vi "Init2.vi"(10 "All_info":string[][](array[string])=[["COM", "COM10", "", ""], ["Save Data", "C:\\AC-BarCode\\Save Data\\", "", ""], ["Model", "C:\\AC-BarCode\\Setting Data\\Model.csv", "", ""], ["CheckPars", "3", "4", "5"], ["LINE", "LINE7", "", ""], ["Title", "三部品照合", "", ""], ["sound", "C:\\AC-BarCode\\sound", "", ""], ["ClearTime", "5", "", ""], ["CheckNum", "3", "", ""], ["LotNo", "11:5", "0:8", "11:8"], ["STANO", "1", "1", "1"], ["WORKNO", "壓縮機", "馬達", "電源板"], ["USEQTY", "1", "1", "1"], ["OPUSER", "SYSTEM", "SYSTEM", "SYSTEM"], ["MMODU", "641", "641", "641"]], 11 "DataIn":T2) -> (3 "DataOut":T2)   [LabVIEW 2014]
uses:
  controls/Data1.ctl
  controls/Payjson.ctl
  controls/Pajson.ctl
panel:
  in  "json 2":T1
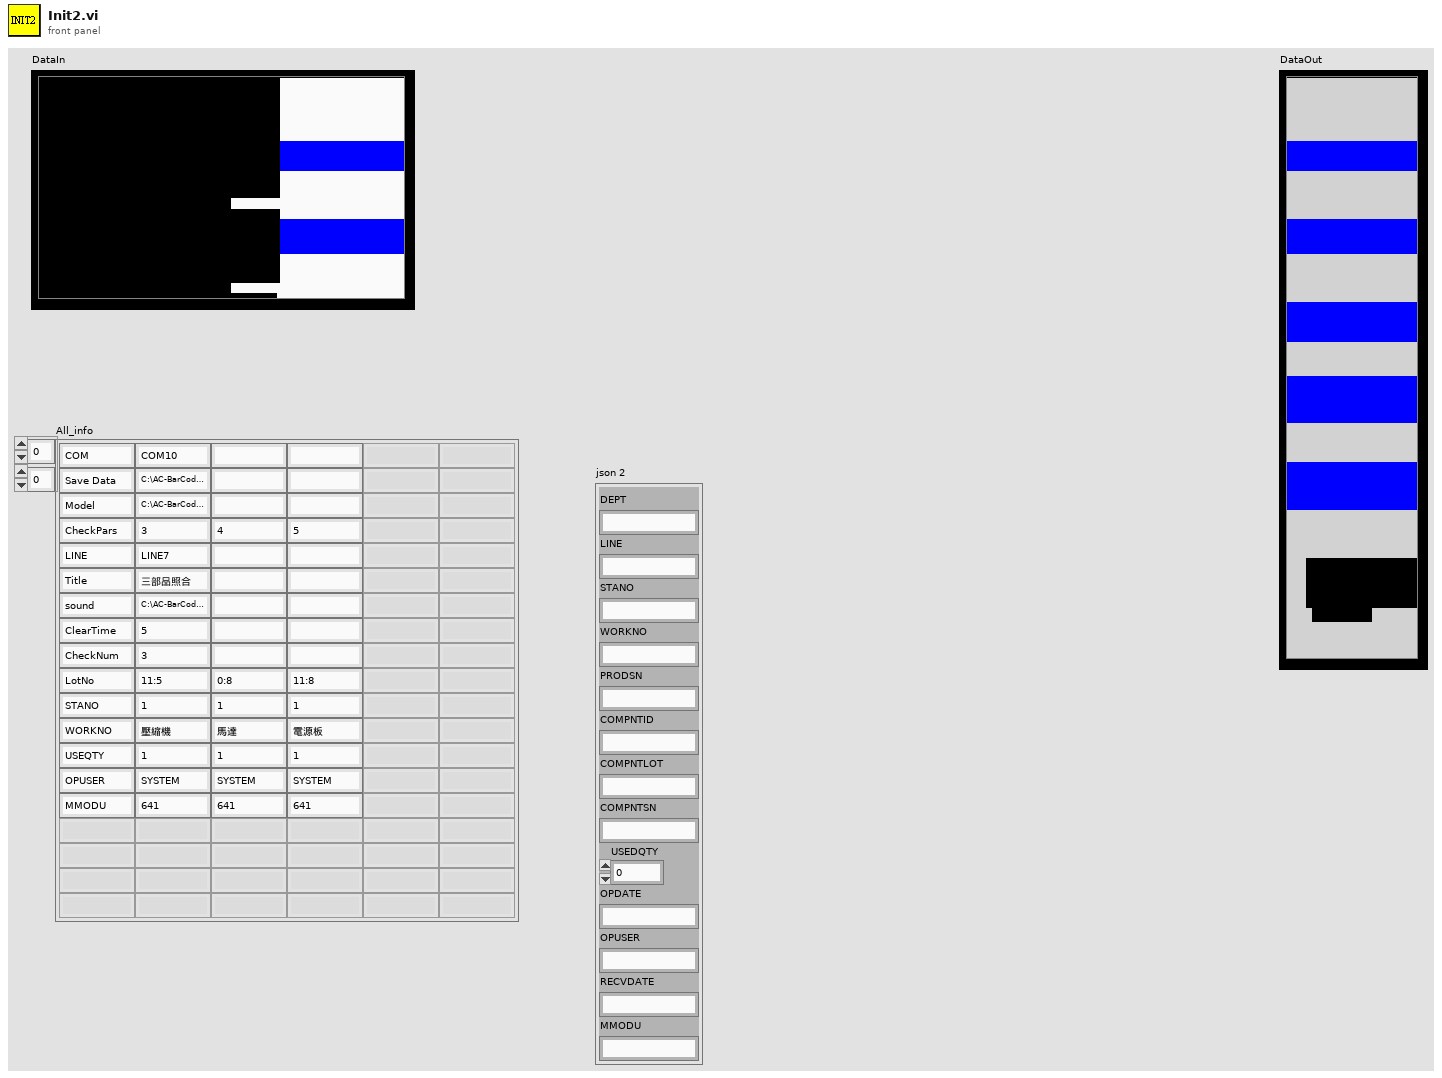
[diagram p1: front panel]
types:
  T1 = typedef "Pajson.ctl" = cluster{"DEPT":string, "LINE":string, "STANO":string, "WORKNO":string, "PRODSN":string, "COMPNTID":string, "COMPNTLOT":string, "COMPNTSN":string, "USEDQTY":i16, "OPDATE":string, "OPUSER":string, "RECVDATE":string, "MMODU":string}
  T2 = typedef "Data1.ctl" = cluster{"Date":string, "BarCode1":string, "BarCode2":string, "BarCode3":string, "Message":string, "OK Count":u16, "NG Count":u16, "Total Count":u16, "ModelData":string[][], "OK&NG":bool, "COM1":refnum<visa-resource-name>, "COM2":refnum<visa-resource-name>, "IO":i32, "Time":u32, "TCP":refnum<k5>, "TCP 2":refnum<k5>, "COM1 2":refnum<visa-resource-name>, "CheckNum":string, "BarCode1_1":string, "BarCode2_1":string, "BarCode3_1":string, "日期":string, "機種":string, "機號":string, "商品條碼1":string, "OK_1":string, "OK":string, "NG":string, "NG_1":string, "Total":string, "Total_1":string, "ClaerTime":u32, "Pjson":T3, "LotNo":string[], "CheckParsArray":string[], "BarCode4":string, "BarCode4_1":string, "商品條碼2":string, "BarCode5":string, "BarCode5_1":string, "商品條碼3":string, "ReScanNG":i32, "NGTimeCT":u32}
  T3 = typedef "Payjson.ctl" = cluster{"DEPT":string, "LINE":string, "STANO":string, "WORKNO":string, "PRODSN":string, "COMPNTID":string, "COMPNTLOT":string, "COMPNTSN":string, "USEDQTY":i16, "OPDATE":string, "OPUSER":string, "RECVDATE":string, "MMODU":string}[]
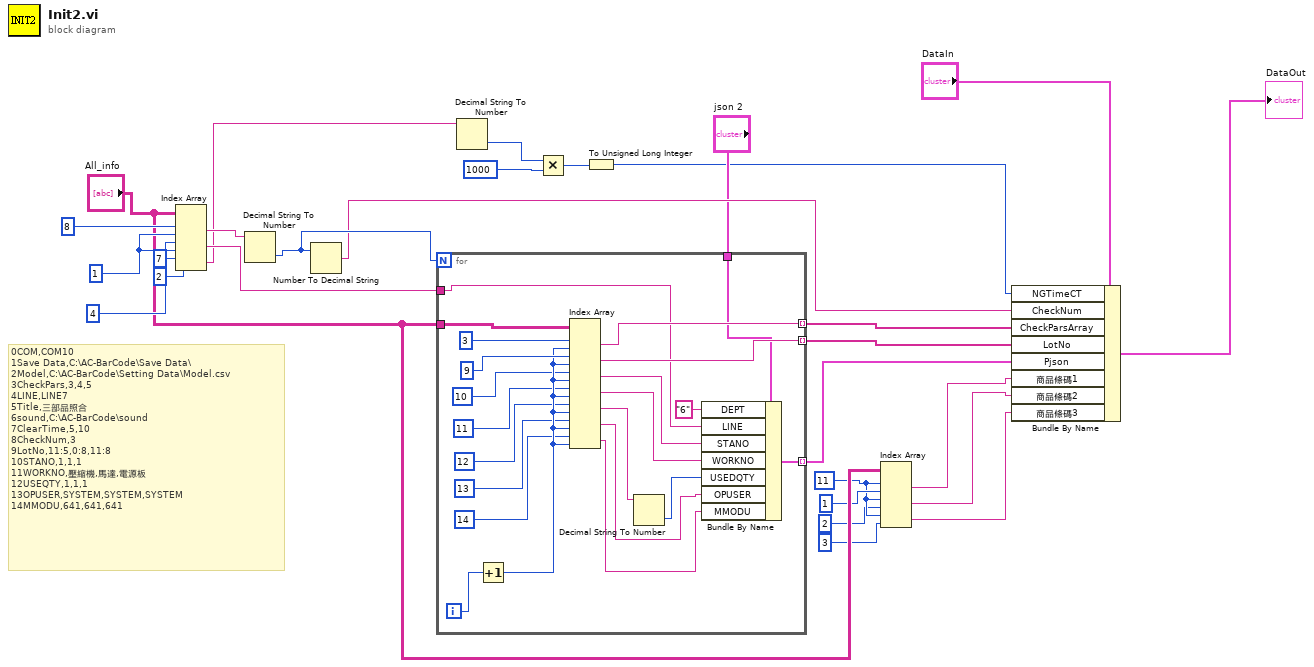
[diagram p0: block diagram]
diagram:
  w13 = 11 ("index (row)")
  w22 = 1 ("disabled index (col)")
  # "0COM,COM10\n1Save Data,C:\\AC-BarCode\\Save Data\\\n2Model,C:\\AC-BarCode\\Setting Data\\Model.csv\n3CheckPars,3,4,5\n4LINE,LINE7\n5Title,三部品照合\n6sound,C:\\AC-BarCode\\sound\n7ClearTime,5,10\n8CheckNum,3\n9LotNo,11:5,0:8,11:8\n10STANO,1,1,1\n11WORKNO,壓縮機,馬達,電源板\n12USEQTY,1,1,1\n13OPUSER,SYSTEM,SYSTEM,SYSTEM\n14MMODU,641,641,641"
  n1 = Index Array(array="All_info", index (row) #1=8 ("disabled index (row)"), index (col) #1=w22, index (row) #2=4 ("disabled index (row)"), index (col) #2=w22, index (row) #3=7 ("index (row)"), index (col) #3=2 ("disabled index (col)")) -> (element #1=w27:string, element #2=w20:string, element #3=w3:string)
  n2 = Decimal String To Number(string=w27) -> (number=w26:i32)  [unwired: 2 in, 1 out]
  n3 = Number To Decimal String(number=w26) -> (decimal integer string=w25:string)  [unwired: 1 in]
  n4 = for {
    N: w26 -> [_]
    tunnel: "All_info" -> [w50]
    tunnel: [w40] -> w24 mode=indexing
    tunnel: [w39] -> w23 mode=indexing
    tunnel: w20 -> [w36]
    tunnel: "json 2" -> [w38]
    tunnel: [w29] -> w18 mode=indexing
    i -> [w49]
    n5 = Increment(x=w49) -> (x+1=w46:i32)
    n6 = Index Array(array=w50, index (row) #1=3 ("disabled index (row)"), index (col) #1=w46, index (row) #2=9 ("disabled index (row)"), index (col) #2=w46, index (row) #3=10 ("disabled index (row)"), index (col) #3=w46, index (row) #4=11 ("disabled index (row)"), index (col) #4=w46, index (row) #5=12 ("disabled index (row)"), index (col) #5=w46, index (row) #6=13 ("disabled index (row)"), index (col) #6=w46, index (row) #7=14 ("disabled index (row)"), index (col) #7=w46) -> (element #1=w40:string, element #2=w39:string, element #3=w35:string, element #4=w34:string, element #5=w33:string, element #6=w31:string, element #7=w30:string)
    n7 = Decimal String To Number(string=w33) -> (number=w32:i32)  [unwired: 2 in, 1 out]
    n8 = Bundle By Name(cluster=w38, "DEPT"="6", "LINE"=w36, "STANO"=w35, "WORKNO"=w34, "USEDQTY"=w32, "OPUSER"=w31, "MMODU"=w30) -> (w29:T1)
  }
  n9 = Decimal String To Number(string=w3) -> (number=w5:i32)  [unwired: 2 in, 1 out]
  n10 = Multiply(x=w5, y=1000) -> (x*y=w1:i32)
  n11 = To Unsigned Long Integer(number=w1) -> (unsigned 32bit integer=w2:u32)
  n12 = Index Array(array="All_info", index (row) #1=w13, index (col) #1=1 ("disabled index (col)"), index (row) #2=w13, index (col) #2=2 ("disabled index (col)"), index (row) #3=w13, index (col) #3=3 ("disabled index (col)")) -> (element #1=w10:string, element #2=w9:string, element #3=w8:string)
  n13 = Bundle By Name(cluster="DataIn", "NGTimeCT"=w2, "CheckNum"=w25, "CheckParsArray"=w24, "LotNo"=w23, "Pjson"=w18, "商品條碼1"=w10, "商品條碼2"=w9, "商品條碼3"=w8) -> (→"DataOut":T2)
